vi "AuMT8852B Continue After Self-Test.vi"(8 "error in (no error)":errorcluster, 11 "VISA session":refnum<visa-resource-name>) -> (0 "error out":errorcluster, 2 "error code":i32, 3 "VISA session out":refnum<visa-resource-name>)   [LabVIEW 2017]
doc: "Anritsu MT8852B Bluetooth Tester\n\nContinues starting up after any error except a DSP error."
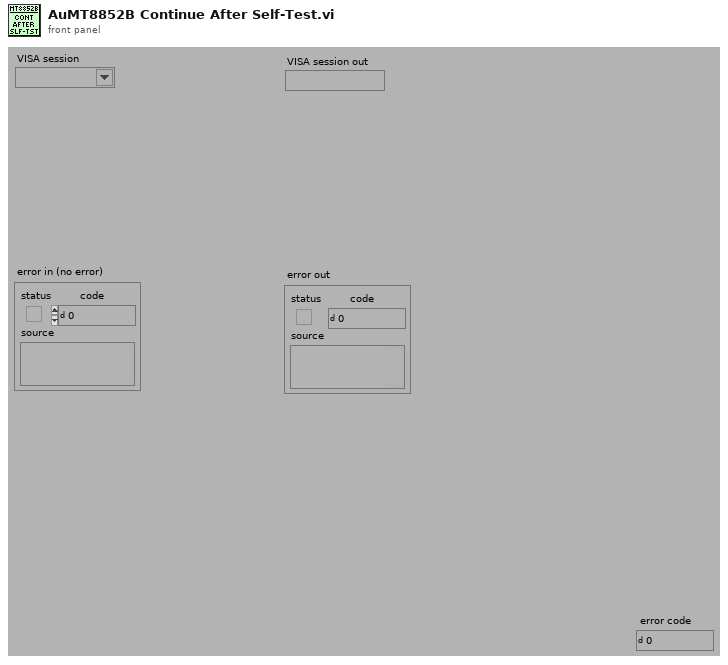
[diagram p1: front panel]
types:
  T1 = enum16{"Simulate", "Range check", "Cache", "Query instrument status"}
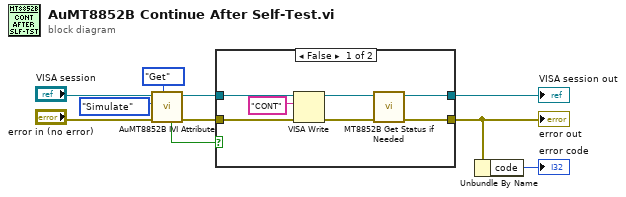
[diagram p0: block diagram]
diagram:
  n1 = call <instrlib>:"AuMT8852B IVI Attribute.vi"("Set/Get (Set)"=enum16{"Set", "Get"}."Get", "error in (no error)"="error in (no error)", "Flag (Simulate)"=T1."Simulate", "VISA session"="VISA session") -> ("error out"=w6:errorcluster, "VISA session out"=w7:refnum<visa-resource-name>, "Value out"=w3:bool)  [unwired: 5 in]
  n2 = case shown="False" w3 {
    tunnel: [w14 w18] -> w1
    tunnel: [w15 w19] -> w8
    tunnel: w7 -> [w17 w19]
    tunnel: w6 -> [w16 w18]
    frame False {
      n3 = VISA Write(VISA resource name=w17, write buffer="CONT" ("write buffer (\"\")"), error in (no error)=w16) -> (VISA resource name out=w12:refnum<visa-resource-name>, error out=w11:errorcluster)  [unwired: 1 out]
      n4 = call <instrlib>:"MT8852B Get Status if Needed.vi"("error in (no error)"=w11, "VISA session"=w12) -> ("error out"=w14:errorcluster, "VISA session out"=w15:refnum<visa-resource-name>)  [unwired: 8 in]
    }
    frame True {
    }
  }
  "error out" <- w1
  "VISA session out" <- w8
  n5 = Unbundle By Name(w1) -> ("code"=→"error code":i32)
